vi "Simple Put Buffer.vi"(0 "remote file uri":string, 1 "username":string, 2 "password":string, 7 "data":string, 11 "error in (no error)":errorcluster) -> (15 "error out":errorcluster)   [LabVIEW 2017, in "NI_WebDAV.lvlib"]
doc: "Uploads a file or multiple files to a remote WebDAV server or target. You must manually select the polymorphic instance you want to use."
uses:
  <vilib>/WebDAVClient/NI_WebDAV.lvlib
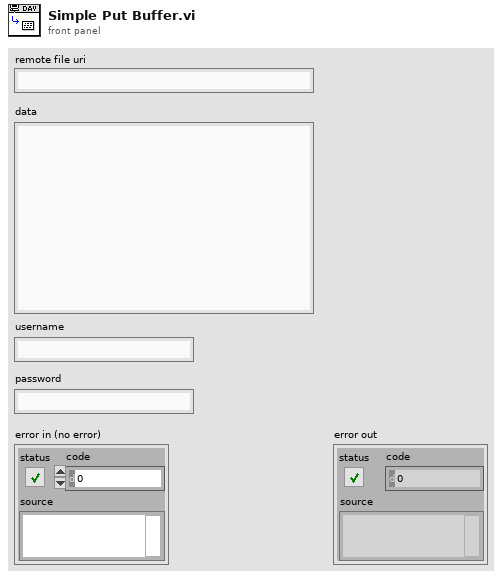
[diagram p1: front panel]
types:
  T1 = typedef "NI_WebDAV.lvlib/SessionHandle.ctl" = refnum<k1>
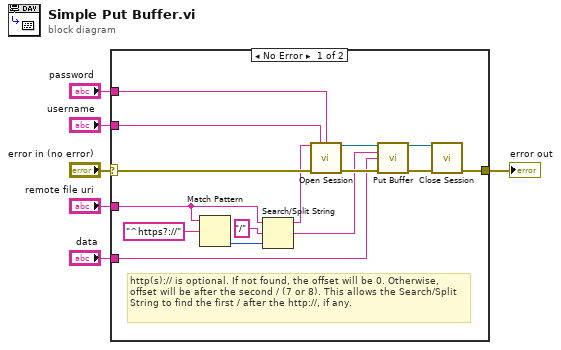
[diagram p0: block diagram]
diagram:
  n1 = case shown="No Error" "error in (no error)" {
    selector: "error in (no error)" -> [w21 w22]
    tunnel: "username" -> [w20 _]
    tunnel: "password" -> [w19 _]
    tunnel: "remote file uri" -> [w9 _]
    tunnel: "data" -> [w16 _]
    tunnel: [w13 w22] -> w1
    frame No Error {
      # "http(s):// is optional. If not found, the offset will be 0. Otherwise, offset will be after the second / (7 or 8). This allows the Search/Split String to find the first / after the http://, if any."
      n2 = Match Pattern(string=w9, regular expression="^https?://") -> (offset past match=w12:i32)  [unwired: 1 in, 3 out]
      n3 = Search/Split String(string=w9, search string/char (-)="/", offset (0)=w12) -> (substring before match=w8:string, match + rest of string=w7:string)  [unwired: 1 out]
      n4 = call <vilib>:"Open Session.vi"("host uri prefix"=w8, "username"=w20, "password"=w19, "error in (no error)"=w21) -> ("session handle out"=w17:T1, "error out"=w18:errorcluster)  [unwired: 10 in]
      n5 = call <vilib>:"Put Buffer.vi"("session handle"=w17, "relative uri"=w7, "data"=w16, "error in (no error)"=w18) -> ("session handle out"=w14:T1, "error out"=w15:errorcluster)  [unwired: 10 in]
      n6 = call <vilib>:"Close Session.vi"("session handle"=w14, "error in (no error)"=w15) -> ("error out"=w13:errorcluster)  [unwired: 13 in]
    }
    frame Error {
    }
  }
  "error out" <- w1
